vi "example test.vi"() -> ()   [LabVIEW 2013, in "EthernetIP tests.lvlib"]
uses:
  EthernetIP tests.lvlib
  configuration/EthernetIP configuration.lvclass
  execution/EthernetIP runtime.lvclass
  <vilib>/NI/Tag Bus/tag/Data Type.ctl
  configuration/assembly type.ctl
  <vilib>/NI/Tag Bus/dictionary/data dictionary.lvclass/data dictionary.ctl
  <vilib>/NI/Tag Bus/dictionary/lookup polymorphs/locate U8.vi
  <vilib>/NI/Tag Bus/table/data polymorphs/write one/write U8.vi
  <vilib>/NI/Tag Bus/table/data polymorphs/read one/read U8.vi
  <vilib>/NI/Tag Bus/dictionary/search/find data index.vi
  <vilib>/NI/Tag Bus/dictionary/search/search string list.vi
  <vilib>/NI/Tag Bus/dictionary/tag not found.vi
  <vilib>/NI/Tag Bus/tag/tag descriptor.lvclass
  <vilib>/NI/Tag Bus/dictionary/data dictionary.lvclass
  <vilib>/NI/Tag Bus/table/data table.lvlib
  channel/EthernetIP Channel.lvclass
panel:
  in  "stop":bool
  in  "value TX":u8(slide)=42 scale=0.0..255.0
  out "value RX":u8(slide) scale=0.0..255.0
  out "final error":errorcluster
  out "output error":errorcluster
  out "input error":errorcluster
  out "output lookup error":errorcluster
  out "no data written":bool
  out "input lookup error":errorcluster
  out "init error":errorcluster
  out "correct execution settings":bool
  out "serialization problem":errorcluster
  out "invalid configuration":errorcluster
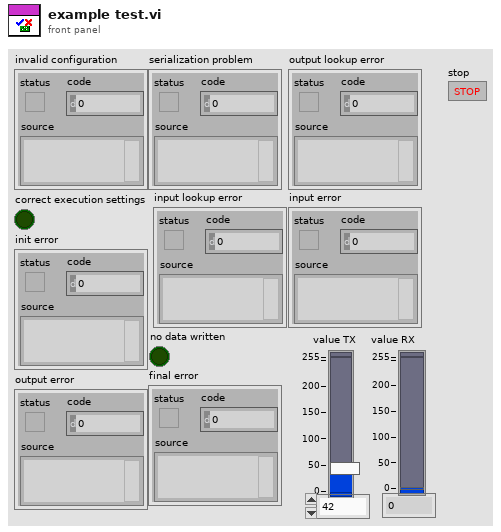
[diagram p1: front panel]
types:
  T1 = typedef "EthernetIP configuration.lvclass/assembly type.ctl" = enum32{"Producing", "Consuming"}
  T2 = typedef "tag bus.lvlib/tag descriptor.lvclass/Data Type.ctl" = enum16{"Double", "Single", "I64", "I32", "I16", "I8", "U64", "U32", "U16", "U8", "Boolean", "String", "Array of Double", "Array of Single", "Array of I64", "Array of I32", "Array of I16", "Array of I8", "Array of U64", "Array of U32", "Array of U16", "Array of U8", "Array of Boolean", "Array of String"}
  T3 = typedef "TBM channel.lvclass/data tables.ctl" = cluster{"input data":T4, "processing parameter":T4, "processing result":T4, "output data":T4}
  T4 = typedef "tag bus.lvlib/dictionary table pair.ctl" = cluster{"data dictionary":refnum<class "data dictionary.lvclass">, "data table":T5}
  T5 = typedef "tag bus.lvlib/data table.lvlib/data table.ctl" = cluster{"Double":dbl[], "Single":sgl[], "I64":i64[], "I32":i32[], "I16":i16[], "I8":i8[], "U64":u64[], "U32":u32[], "U16":u16[], "U8":u8[], "Boolean":bool[], "String":string[], "Array of Double":cluster{"DBL Array":dbl[]}[], "Array of Single":cluster{"SGL Array":sgl[]}[], "Array of I64":cluster{"I64 Array":i64[]}[], "Array of I32":cluster{"I32 Array":i32[]}[], "Array of I16":cluster{"I16 Array":i16[]}[], "Array of I8":cluster{"I8 Array":i8[]}[], "Array of U64":cluster{"U64 Array":u64[]}[], "Array of U32":cluster{"U32 Array":u32[]}[], "Array of U16":cluster{"U16 Array":u16[]}[], "Array of U8":cluster{"U8 Array":u8[]}[], "Array of Boolean":cluster{"Boolean Array":bool[]}[], "Array of String":cluster{"String Array":string[]}[]}
  T6 = typedef "TBM module execution interface.lvclass/execution settings.ctl" = cluster{"reads inputs":bool, "processes data":bool, "writes outputs":bool}
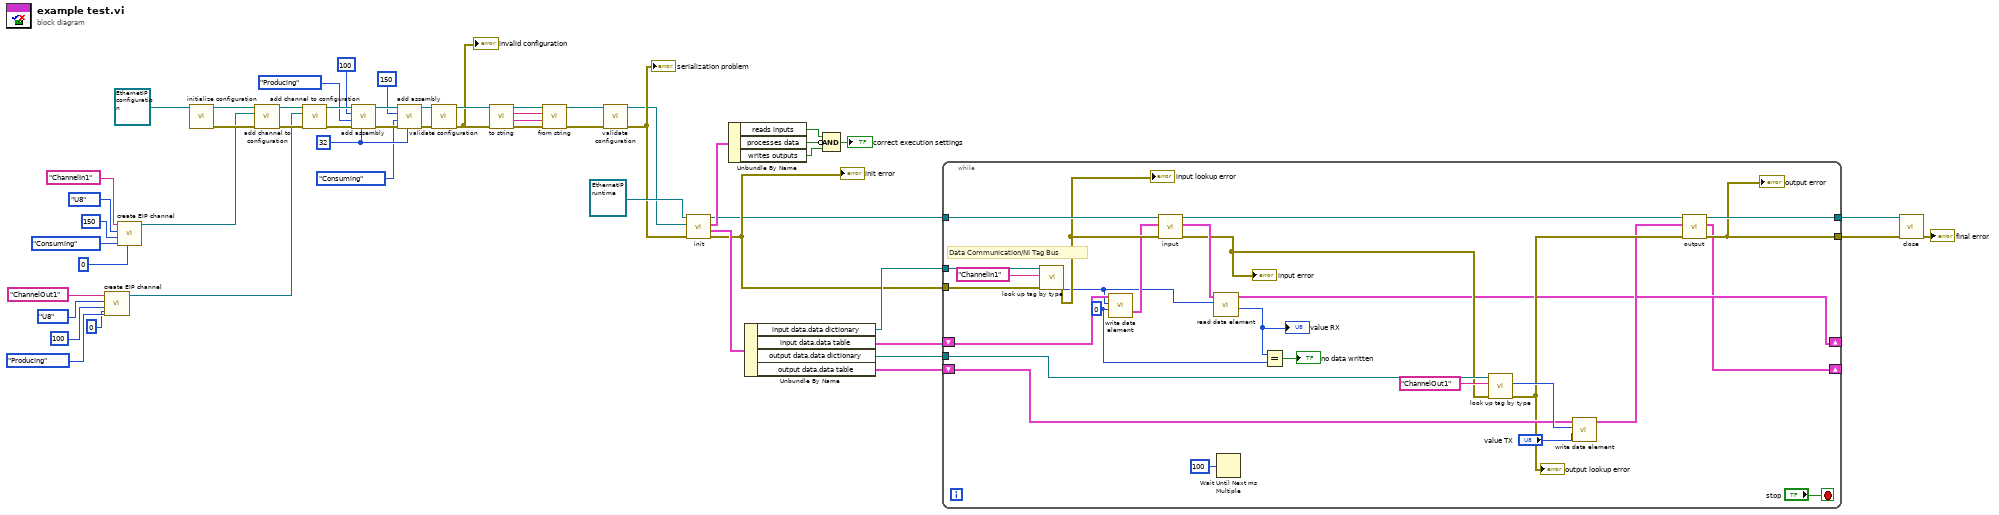
[diagram p0: block diagram]
diagram:
  w5 = u32 32 ("Size (bytes)")
  n1 = call "create EIP channel.vi"("byte index"=0, "Type"=assembly_type."Producing", "Instance ID"=u32 100, "data type"=Data_Type."U8", "name"="ChannelOut1" ("channel name")) -> ("EthernetIP Channel out"=w16:refnum<class "EthernetIP Channel.lvclass">)  [unwired: 6 in]
  n2 = call "create EIP channel.vi"("byte index"=0, "Type"=assembly_type."Consuming", "Instance ID"=u32 150, "data type"=Data_Type."U8", "name"="ChannelIn1" ("channel name")) -> ("EthernetIP Channel out"=w10:refnum<class "EthernetIP Channel.lvclass">)  [unwired: 6 in]
  n3 = call-dynamic "initialize configuration.vi"("configuration in"=refnum<class "EthernetIP configuration.lvclass"> refnum ("tag bus configurable plugin module configuration")) -> ("error out"=w24:errorcluster, "configuration out"=w25:refnum<class "EthernetIP configuration.lvclass">)  [unwired: 8 in, 1 out]
  n4 = call "add channel to configuration.vi"("error in"=w24, "TBM channel in"=w10, "EthernetIP configuration in"=w25) -> ("error out"=w26:errorcluster, "EthernetIP configuration out"=w27:refnum<class "EthernetIP configuration.lvclass">)  [unwired: 7 in]
  n5 = call "add channel to configuration.vi"("error in"=w26, "TBM channel in"=w16, "EthernetIP configuration in"=w27) -> ("error out"=w23:errorcluster, "EthernetIP configuration out"=w8:refnum<class "EthernetIP configuration.lvclass">)  [unwired: 7 in]
  n6 = call "add assembly.vi"("size (bytes)"=w5, "error in"=w23, "Type"=assembly_type."Producing", "instance ID"=u32 100 ("Instance ID"), "EthernetIP configuration in"=w8) -> ("error out"=w9:errorcluster, "EthernetIP configuration out"=w6:refnum<class "EthernetIP configuration.lvclass">)  [unwired: 5 in]
  n7 = call "add assembly.vi"("size (bytes)"=w5, "error in"=w9, "Type"=assembly_type."Consuming", "instance ID"=u32 150 ("Instance ID"), "EthernetIP configuration in"=w6) -> ("error out"=w7:errorcluster, "EthernetIP configuration out"=w22:refnum<class "EthernetIP configuration.lvclass">)  [unwired: 5 in]
  n8 = call-dynamic "validate configuration.vi"("error in"=w7, "EthernetIP configuration in"=w22) -> ("error out"=w53:errorcluster, "EthernetIP configuration out"=w54:refnum<class "EthernetIP configuration.lvclass">)  [unwired: 8 in]
  "invalid configuration" <- w53
  n9 = call-dynamic "to string.vi"("error in"=w53, "EthernetIP configuration in"=w54) -> ("error out"=w49:errorcluster, "data"=w50:string, "version"=w51:string, "EthernetIP configuration out"=w52:refnum<class "EthernetIP configuration.lvclass">)  [unwired: 6 in]
  n10 = call-dynamic "from string.vi"("error in"=w49, "data"=w50, "version"=w51, "EthernetIP configuration in"=w52) -> ("error out"=w47:errorcluster, "EthernetIP configuration out"=w48:refnum<class "EthernetIP configuration.lvclass">)  [unwired: 6 in]
  n11 = call-dynamic "validate configuration.vi"("error in"=w47, "EthernetIP configuration in"=w48) -> ("error out"=w45:errorcluster, "EthernetIP configuration out"=w44:refnum<class "EthernetIP configuration.lvclass">)  [unwired: 8 in]
  "serialization problem" <- w45
  n12 = call-dynamic "init.vi"("error in"=w45, "TBM module configuration in"=w44, "EthernetIP runtime in"=refnum<class "EthernetIP runtime.lvclass"> refnum ("tag bus configurable plugin module")) -> ("error out"=w36:errorcluster, "data allocations"=w38:T3, "execution settings"=w43:T6, "EthernetIP runtime out"=w34:refnum<class "EthernetIP runtime.lvclass">)  [unwired: 5 in]
  "init error" <- w36
  n13 = Unbundle By Name(w43) -> ("reads inputs"=w40:bool, "processes data"=w42:bool, "writes outputs"=w41:bool)
  n14 = Unbundle By Name(w38) -> ("input data.data dictionary"=w37:refnum<class "data dictionary.lvclass">, "input data.data table"=w35:T5, "output data.data dictionary"=w33:refnum<class "data dictionary.lvclass">, "output data.data table"=w32:T5)
  n15 = Compound Arithmetic op=AND(w40, invert w42, w41) -> (→"correct execution settings":bool)
  n16 = while {
    tunnel: w37 -> [w81]
    tunnel: w36 -> [w80]
    tunnel: w34 -> [w77]
    tunnel: w33 -> [w70]
    tunnel: [w61] -> w31
    tunnel: [w60] -> w30
    shift-right: [w57] -> _
    shift-left: w32 -> [w67]
    shift-right: [w58] -> _
    shift-left: w35 -> [w78]
    stop <- "stop" stop-if-true
    w59 = u8 0 ("value")
    # "Data Communication/NI Tag Bus"
    n17 = call-poly <vilib>:"look up tag by type.vi"("error in"=w80, "name"="ChannelIn1" ("channel name"), "data dictionary in"=w81) -> ("error out"=w76:errorcluster, "index"=w73:i32)  [unwired: 6 in, 1 out]
    "input lookup error" <- w76
    n18 = call-poly <vilib>:"write data element.vi"("value"=w59, "index"=w73, "data table in"=w78) -> ("data table out"=w75:T5)  [unwired: 8 in]
    n19 = call-dynamic "input.vi"("error in"=w76, "data table in"=w75, "EthernetIP runtime in"=w77) -> ("error out"=w66:errorcluster, "data table out"=w74:T5, "EthernetIP runtime out"=w63:refnum<class "EthernetIP runtime.lvclass">)  [unwired: 6 in]
    "input error" <- w66
    n20 = call-poly <vilib>:"read data element.vi"("index"=w73, "data table in"=w74) -> ("value"=w72:u8, "data table out"=w58:T5)  [unwired: 8 in]
    "value RX" <- w72
    n21 = Wait Until Next ms Multiple(millisecond multiple=u32 100) -> ()  [unwired: 1 out]
    n22 = Equal?(x=w72, y=w59) -> (x = y?=→"no data written":bool)
    n23 = call-poly <vilib>:"look up tag by type.vi"("error in"=w66, "name"="ChannelOut1" ("channel name"), "data dictionary in"=w70) -> ("error out"=w64:errorcluster, "index"=w68:i32)  [unwired: 6 in, 1 out]
    "output lookup error" <- w64
    n24 = call-poly <vilib>:"write data element.vi"("value"="value TX", "index"=w68, "data table in"=w67) -> ("data table out"=w62:T5)  [unwired: 8 in]
    n25 = call-dynamic "output.vi"("error in"=w64, "data table in"=w62, "EthernetIP runtime in"=w63) -> ("error out"=w60:errorcluster, "data table out"=w57:T5, "EthernetIP runtime out"=w61:refnum<class "EthernetIP runtime.lvclass">)  [unwired: 6 in]
    "output error" <- w60
  }
  n26 = call-dynamic "close.vi"("error in"=w30, "EthernetIP runtime in"=w31) -> ("error out"=→"final error":errorcluster)  [unwired: 9 in]
